vi "Choose Options.vi"(7 "Shared Options":refnum<class "Shared Options.lvclass">, 11 "Local Options":string[](array[string])) -> (3 "Options":string[](array[string]))   [LabVIEW 2020, in "AutoComplete.lvlib"]
uses:
  AutoComplete.lvlib
  Shared Options/Shared Options.lvclass
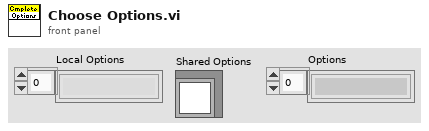
[diagram p1: front panel]
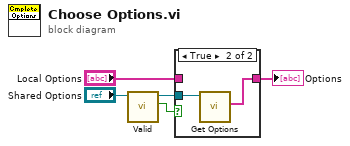
[diagram p0: block diagram]
diagram:
  n1 = call "Valid.vi"("Shared Options in"="Shared Options") -> ("Valid"=w4:bool, "Shared Options out"=w1:refnum<class "Shared Options.lvclass">)  [unwired: 8 in, 1 out]
  n2 = case shown="True" w4 {
    tunnel: "Local Options" -> [w6 _]
    tunnel: [w6 w7] -> w2
    tunnel: w1 -> [_ w8]
    frame False {
    }
    frame True {
      n3 = call "Get Options.vi"("Shared Options in"=w8) -> ("Options"=w7:string[])  [unwired: 8 in, 2 out]
    }
  }
  "Options" <- w2
